vi "Format String tester.vi"() -> ()   [LabVIEW 2010]
panel:
  out "spreadsheet string":string
  in  "delimiter (\\t)":string="\t"
  in  "array":dbl[][](array[numeric])
  in  "format string":string="%#g"
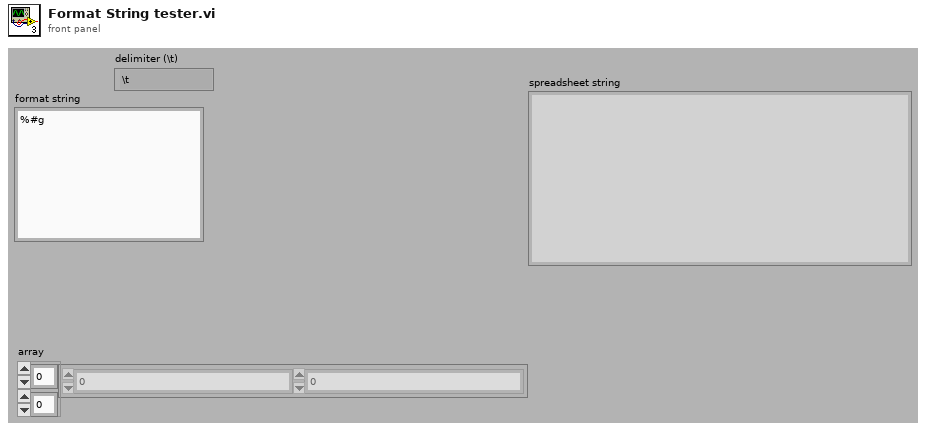
[diagram p1: front panel]
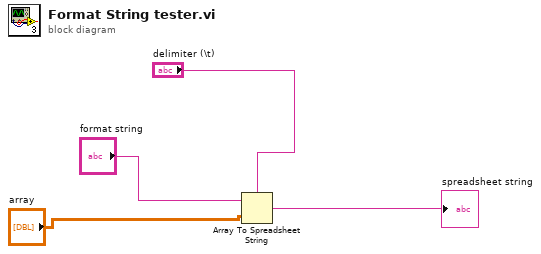
[diagram p0: block diagram]
diagram:
  n1 = Array To Spreadsheet String(delimiter (Tab)="delimiter (\\t)", array="array", 3:"format string") -> (spreadsheet string=→"spreadsheet string":string)
